vi "LSX Set TVR Out Mode.vi"(6 "lRT":i32, 7 "lZT":i32, 8 "error in (no error)":errorcluster, 9 "lYT":i32, 10 "lXT":i32, 11 "lLSID":i32) -> (0 "error out":errorcluster, 3 "function return":i32)   [LabVIEW 2018, in "Tango.lvlib"]
doc: "TANGOAPI int TANGOCALL LSX_SetTVROutMode (int lLSID, int lXT, int lYT, int lZT, int lRT);"
uses:
  <userlib>/Tango/Tango.lvlib
  <userlib>/Tango/Tango_DLL.dll
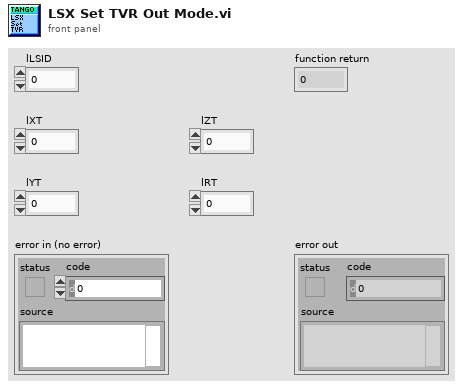
[diagram p1: front panel]
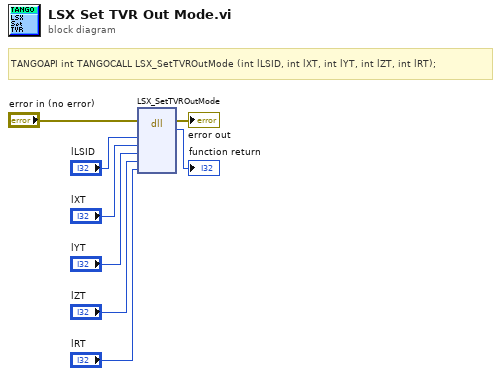
[diagram p0: block diagram]
diagram:
  # "TANGOAPI int TANGOCALL LSX_SetTVROutMode (int lLSID, int lXT, int lYT, int lZT, int lRT);"
  n1 = dll-call lib="C:/Program Files (x86)/National Instruments/LabVIEW 2018/user.lib/Tango/Tango_DLL.*" fn="LSX_SetTVROutMode"(error in="error in (no error)", "lLSID"="lLSID", "lXT"="lXT", "lYT"="lYT", "lZT"="lZT", "lRT"="lRT") -> (error out=→"error out":errorcluster, →"function return":i32)  [unwired: 7 in, 1 out]
